vi "Modify Class Data.vi"(8 "error in (no error)":errorcluster, 11 "QControl Creation in":refnum<class "QControl Creation.lvclass">) -> (0 "error out":errorcluster, 3 "QControl Creation (dup)":refnum<class "QControl Creation.lvclass">)   [LabVIEW 2023, in "QControl Creation.lvclass"]
doc: "<b> </b> <b> </b>\n©2016 Q Software Innovations, LLC (QSI)\nwritten by Quentin Alldredge\nproduced in LabVIEW 2015\n\nsupport@qsoftwareinnovations.com\nwww.qsoftwareinnovations.com\n\nAll rights reserved.\n\nRedistribution and use in source and binary forms, with or without modification, are permitted provided that the following conditions are met:\n\n * Redistributions of source code must retain the above copyright notice, this list of conditions and the following disclaimer.\n * Redistributions in binary form must reproduce the above copyright notice, this list of conditions and the following disclaimer in the documentation and/or other materials provided with the distribution.\n * Neither the name of Q Software Innovations, LLC. nor the names of its contributors may be used to endorse or promote products derived from this software without specific prior written permission.\n\nTHIS SOFTWARE IS PROVIDED BY THE COPYRIGHT HOLDERS AND CONTRIBUTORS \"AS IS\" AND ANY EXPRESS OR IMPLIED WARRANTIES, INCLUDING, BUT NOT LIMITED TO, THE IMPLIED WARRANTIES OF MERCHANTABILITY AND FITNESS FOR A PARTICULAR PURPOSE ARE DISCLAIMED. IN NO EVENT SHALL THE COPYRIGHT OWNER OR CONTRIBUTORS BE LIABLE FOR ANY DIRECT, INDIRECT, INCIDENTAL, SPECIAL, EXEMPLARY, OR CONSEQUENTIAL DAMAGES (INCLUDING, BUT NOT LIMITED TO, PROCUREMENT OF SUBSTITUTE GOODS OR SERVICES; LOSS OF USE, DATA, OR PROFITS; OR BUSINESS INTERRUPTION) HOWEVER CAUSED AND ON ANY THEORY OF LIABILITY, WHETHER IN CONTRACT, STRICT LIABILITY, OR TORT (INCLUDING NEGLIGENCE OR OTHERWISE) ARISING IN ANY WAY OUT OF THE USE OF THIS SOFTWARE, EVEN IF ADVISED OF THE POSSIBILITY OF SUCH DAMAGE."
uses:
  QControl Creation.lvclass
  <vilib>/Utility/miscctls.llb/LVPositionTypeDef.ctl
  QControl Creation.lvclass/QControl Creation.ctl
  <vilib>/Utility/error.llb/Error Cluster From Error Code.vi
  <vilib>/ErrorRing/Error Ring.xnode
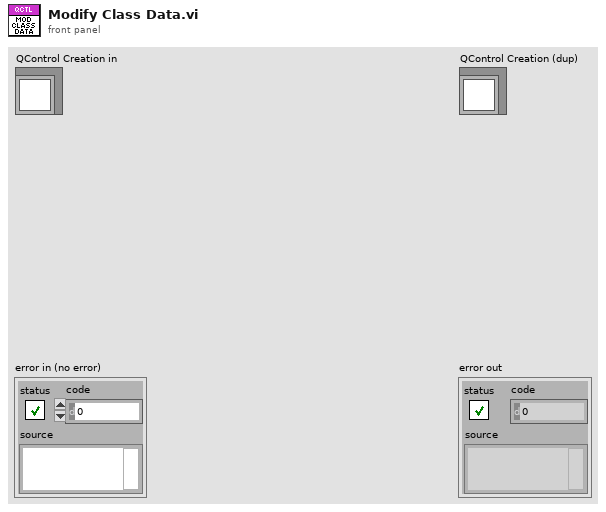
[diagram p1: front panel]
types:
  T1 = typedef "LVPositionTypeDef.ctl" = cluster{"Left":i32, "Top":i32}
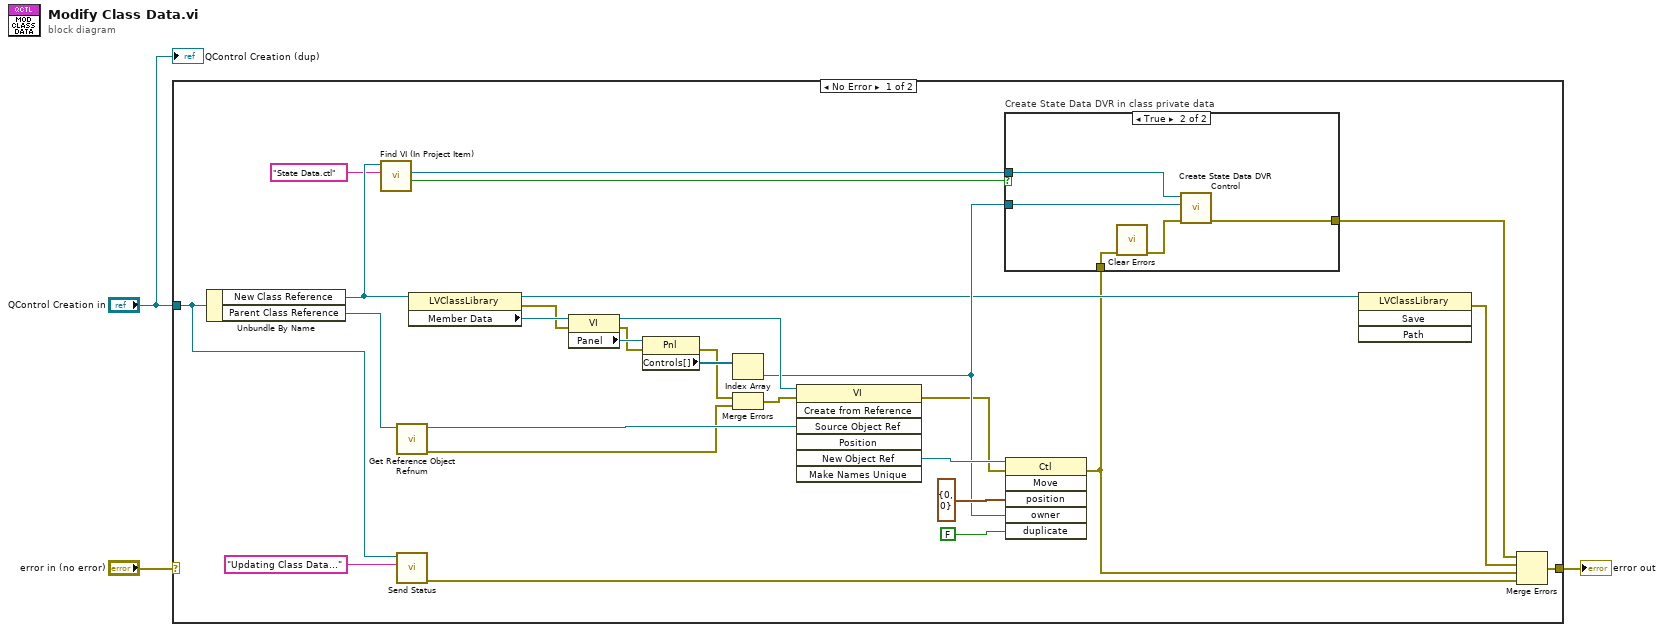
[diagram p0: block diagram]
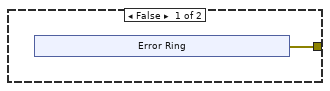
[diagram p2: hidden frame]
diagram:
  n1 = case shown="No Error" "error in (no error)" {
    selector: "error in (no error)" -> [_ w43]
    tunnel: [w29 w43] -> w2
    tunnel: "QControl Creation in" -> [w9 _]
    frame No Error {
      n2 = Unbundle By Name(w9) -> ("New Class Reference"=w17:refnum<vi>, "Parent Class Reference"=w27:refnum<vi>)
      n3 = call "Find VI (In Project Item).vi"("VI Name"="State Data.ctl", "ProjectItem in"=w17) -> ("Found?"=w8:bool, "VI ProjectItem Refnum"=w15:refnum<vi>)  [unwired: 7 in, 1 out]
      n4 = call "Get Reference Object Refnum.vi"("LVClassLibrary in"=w27) -> ("error out"=w5:errorcluster, "LVObjectRefNum out"=w26:refnum<vi>)  [unwired: 8 in, 1 out]
      n5 = call "Send Status.vi"("Status"="Updating Class Data..." ("Add Item"), "QControl Creation in"=w9) -> ("error out (dup)"=w10:errorcluster)  [unwired: 8 in, 1 out]
      n6 = property class="LVClassLibrary"(reference=w17) -> (reference out=w20:refnum<vi>, error out=w14:errorcluster, "Member Data"=w31:refnum<vi>)  [unwired: 1 in]
      n7 = property class="VI"(reference=w31, error in=w14) -> (reference out=w25:refnum<vi>, error out=w13:errorcluster, "Panel"=w28:refnum<vi>)
      n8 = property class="Pnl"(reference=w28, error in=w13) -> (error out=w12:errorcluster, "Controls[]"=w30:refnum<vi>[])  [unwired: 1 out]
      n9 = Index Array(array=w30) -> (element=w21:refnum<vi>)  [unwired: 1 in]
      n10 = Merge Errors(w12, w5) -> (w6:errorcluster)
      n11 = invoke class="VI" method="Create from Reference"(reference=w25, error in=w6, "Source Object Ref"=w26) -> (error out=w18:errorcluster, "New Object Ref"=w22:refnum<vi>)  [unwired: 4 in, 5 out]
      n12 = invoke class="Ctl" method="Move"(reference=w22, error in=w18, "position"=T1 {"Left"=0, "Top"=0}, "owner"=w21, "duplicate"=FALSE ("Duplicate? (F)")) -> (error out=w4:errorcluster)  [unwired: 1 in, 5 out]
      n13 = case "Create State Data DVR in class private data" shown="True" w8 {
        tunnel: w21 -> [_ w42]
        tunnel: [w32 w41] -> w7
        tunnel: w15 -> [_ w38]
        tunnel: w4 -> [_ w40]
        frame False {
          n14 = xnode "Error Ring"() -> ("error out"=w32:errorcluster)
        }
        frame True {
          n15 = call <vilib>:"Clear Errors.vi"("error in (no error)"=w40) -> ("error out"=w39:errorcluster)  [unwired: 5 in, 1 out]
          n16 = call "Create State Data DVR Control.vi"("error in (no error)"=w39, "Private Data Cluster Control"=w42, "State Data.ctl ProjectIItem"=w38) -> ("error out"=w41:errorcluster)  [unwired: 8 in]
        }
      }
      n17 = invoke class="LVClassLibrary" method="Save"(reference=w20) -> (error out=w19:errorcluster)  [unwired: 3 in, 3 out]
      n18 = Merge Errors(w7, w19, w4, w10) -> (w29:errorcluster)
    }
    frame Error {
    }
  }
  "error out" <- w2
  "QControl Creation (dup)" <- "QControl Creation in"
